vi "9-Move or Create File.vi"() -> ()   [LabVIEW 2020]
uses:
  <vilib>/Utility/sysdir.llb/System Directory Type.ctl
panel:
  out "File exists":bool
  in  "Name or relative path to move file":path
  out "Full Target Path(where the file has been moved)":path
  out "An error occured":bool
  out "error out":errorcluster
  in  "error in (no error)":errorcluster
  out "File doesn't exist but created":bool
  out "File Exists and Moved":bool
  out "File Path":path
  out "folder names":string[](array[string])
  in  "File Name":string
  out "filenames":string[](array[string])
  in  "Search Location":path
  # "The user can list folders and files in the desired location by just entering a path to\n\"Search Location\" line and rrunning the program.(Error indicator should be considered when moving or creating a file the file so user can ignore it when using listing). For creating a nonexisting file in a in the desired location,  type a file name in \"File Name\" line. In order to move a file to a desired location, firstly file should exists,\nthen path to be moved to must be typed in."
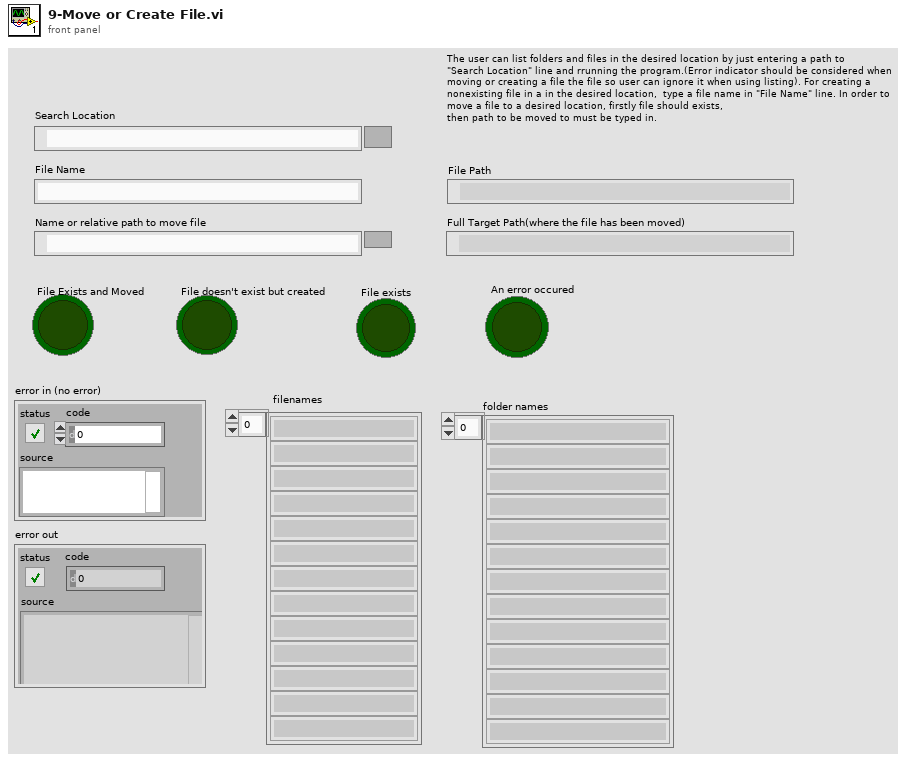
[diagram p1: front panel]
types:
  T1 = typedef "System Directory Type.ctl" = i32
  T2 = enum16{"open", "replace", "create", "open or create", "replace or create", "replace or create with confirmation"}
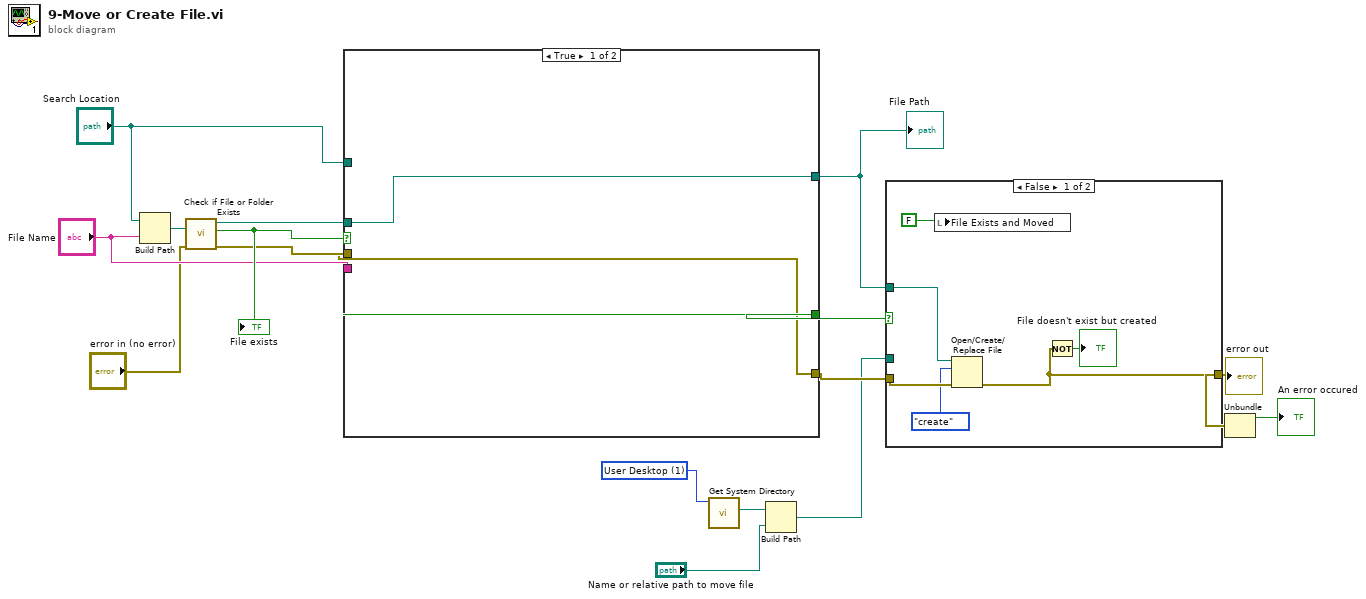
[diagram p0: block diagram]
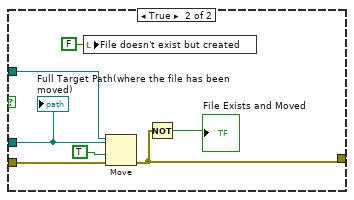
[diagram p2: hidden frame]
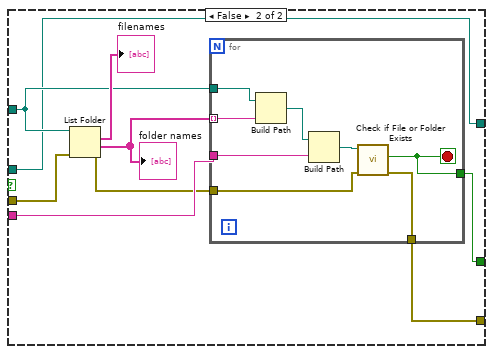
[diagram p3: hidden frame]
diagram:
  w11 = T1 1 items=["User Home"=0, "User Desktop"=1, "User Documents"=2, "User Application Data"=3, "User Preferences"=4, "User Temporary"=5, "Public Documents"=6, "Public Application Data"=7, "Public Preferences"=8, "Public Cache"=13, "System Core Libraries"=9, "System Installed Libraries"=10, "Application Files"=11, "Boot Volume Root"=12] ("system directory type")
  n1 = Build Path(base path="Search Location", name or relative path="File Name") -> (appended path=w16:path)
  n2 = call <vilib>:"Check if File or Folder Exists.vi"("error in (no error)"="error in (no error)", "path"=w16) -> ("error out"=w7:errorcluster, "file or folder exists?"=w15:bool, "dup path"=w14:path)  [unwired: 7 in]
  "File exists" <- w15
  n3 = case shown="True" w15 {
    selector: w15 -> [w19 _]
    tunnel: "File Name" -> [_ w26]
    tunnel: [w18 w20] -> w12
    tunnel: [w19 w24] -> w13
    tunnel: w14 -> [w18 w20]
    tunnel: w7 -> [w17 w23]
    tunnel: [w17 w25] -> w6
    tunnel: "Search Location" -> [_ w21]
    frame True {
    }
    frame False {
      n4 = List Folder(path=w21, error in=w23) -> (filenames=→"filenames":string[], folder names=w27:string[], error out=w22:errorcluster)  [unwired: 2 in, 1 out]
      "folder names" <- w27
      n5 = for {
        tunnel: w27 -> [w32] mode=indexing
        tunnel: w21 -> [w35]
        tunnel: w26 -> [w34]
        tunnel: [w31] -> w25
        tunnel: [w30] -> w24
        tunnel: w22 -> [w29]
        stop <- w30 stop-if-true
        n6 = Build Path(base path=w35, name or relative path=w32) -> (appended path=w36:path)
        n7 = Build Path(base path=w36, name or relative path=w34) -> (appended path=w33:path)
        n8 = call <vilib>:"Check if File or Folder Exists.vi"("error in (no error)"=w29, "path"=w33) -> ("error out"=w31:errorcluster, "file or folder exists?"=w30:bool)  [unwired: 7 in, 1 out]
      }
    }
  }
  "File Path" <- w12
  n9 = call <vilib>:"Get System Directory.vi"("system directory type"=w11) -> ("system directory"=w10:path)  [unwired: 10 in]
  n10 = Build Path(base path=w10, name or relative path="Name or relative path to move file") -> (appended path=w3:path)
  n11 = case shown="False" w13 {
    tunnel: w12 -> [w37 w49]
    tunnel: w3 -> [_ w44]
    tunnel: w6 -> [w42 w48]
    tunnel: [w38 w46] -> w5
    frame False {
      n12 = local write "File Exists and Moved"(FALSE) -> ()
      n13 = Open/Create/Replace File(file path (use dialog)=w37, error in=w42, operation (0:open)=T2."create") -> (error out=w38:errorcluster)  [unwired: 3 in, 2 out]
      n14 = Not(x=w38) -> (.not. x?=→"File doesn't exist but created":bool)
    }
    frame True {
      n15 = local write "File doesn't exist but created"(FALSE ("File Exists and Moved")) -> ()
      n16 = Move(source path=w49, error in=w48, 9:TRUE ("overwrite (F)"), 10:w44) -> (error out=w46:errorcluster)  [unwired: 1 in, 2 out]
      n17 = Not(x=w46) -> (.not. x?=→"File Exists and Moved":bool)
      "Full Target Path(where the file has been moved)" <- w44
    }
  }
  "error out" <- w5
  n18 = Unbundle(w5) -> ("status"=→"An error occured":bool)  [unwired: 2 out]
